vi "GEA3 HEWH Parse ERD.vi"(4 "Enable Heat Pump List":bool, 6 "Enable EMV List?":bool, 8 "Error In":errorcluster, 11 "ERD Data Out":T3[](array[typedef]) {"ERD Number" format="%.0x"}) -> (0 "Error Out":errorcluster, 2 "ERD Data":string[][](array[string]), 3 "ERD Data":T1)   [LabVIEW 2019]
uses:
  type defs/ERD Read Data Out.ctl
  Type Definitions/GEA3 HEWH ERD Data.ctl
  Type Definitions/GEA3 HEWH Mixing Valve.ctl
  library/GEA2_Toolkit.lvlib
panel:
  out "ERD Headers":string[](array[string])=["APPLIANCE SOFTWARE VERSION (0x0100)", "USER SET MODE (0X4020)", "OPERATING MODE (0X4021)", "USER SETPOINT (0x4024)", "ACTUAL SETPOINT (0x4026)", "MODEL DESIGNATOR (0x4042)", "DLB RELAY (0x4068)", "COMPRESSOR RELAY (0x4068)", "LOWER ELEMENT RELAY (0x4068)", "UPPER ELEMENT RELAY (0x4068)", "FAN (0x4068)", "T1 TEMP (0x405F)", "T2 TEMP (0x4060)", "T3A TEMP (0x4061)", "T3B TEMP (0x4062)", "T4 TEMP (0x4063)", "T5 TEMP (0x4064)", "VOLTAGE (0x4066)", "DLB CURRENT (0x4065)", "EEV POSITION (0x4067)", "FLOW EVENTS (0x4069)", "STORED THERMAL CAPACITANCE (0x4058)", "AVAILABLE THERMAL CAPACITANCE (0x4059)", "MAXIMUM THERMAL CAPACITANCE (0X405A)", "NEEA MODE ENABLED (0X404F)", "TANK SIZE (0X4041)", "MIXING VALVE THERMAL CAPACITY SETTING (0X4029)", "T6 TEMP (0x406E)", "T7 TEMP (0x407D)", "MIX VALVE STEP OFFSET (0x4072)", "MIX VALVE STEP ABSOLUTE (0x4073)", "TANK TCO STATE (0x4074)", "OUTLET TCO STATE (0x4075)", "FLOW (0x407E)", "MANUAL (0x407F)", "TANK SETPOINT (0x4078)", "MIX VALVE DELTA T (0x4077)", "PID OUTPUT POSITION (0x407C)", "DAY 1 COLDEST SUPPLY (0x40B0)", "DAY 2 COLDEST SUPPLY (0x40B1)", "DAY 3 COLDEST SUPPLY (0x40B2)", "DAY 4 COLDEST SUPPLY (0x40B3)", "DAY 5 COLDEST SUPPLY (0x40B4)", "DAY 6 COLDEST SUPPLY (0x40B5)", "DAY 7 COLDEST SUPPLY (0x40B6)", "SUPPLY TEMP (0x40B7)", "FIRST STAGE KP GAIN (0xF011)", "FIRST STAGE KI GAIN (0xF012)", "FIRST STAGE KD GAIN (0xF013)", "FIRST STAGE KPQ BITS (0xF014)", "FIRST STAGE KI BITS (0xF015)", "FIRST STAGE KDQ BITS (0xF016)", "SECOND STAGE KP GAIN (0xF021)", "SECOND STAGE KI GAIN (0xF022)", "SECOND STAGE KD GAIN (0xF023)", "SECOND STAGE KPQ BITS (0xF024)", "SECOND STAGE KIQ BITS (0xF025)", "SECOND STAGE KDQ BITS (0xF026)", "THIRD STAGE KP GAIN (0xF031)", "THIRD STAGE KI GAIN (0xF032)", "THIRD STAGE KD GAIN (0xF033)", "THIRD STAGE KPQ BITS (0xF034)", "THIRD STAGE KIQ BITS (0xF035)", "THIRD STAGE KDQ BITS (0xF036)", "FOURTH STAGE KP GAIN (0xF041)", "FOURTH STAGE KI GAIN (0xF042)", "FOURTH STAGE KD GAIN (0xF043)", "FOURTH STAGE KPQ BITS (0xF044)", "FOURTH STAGE KIQ BITS (0xF045)", "FOURTH STAGE KDQ BITS (0xF046)"]
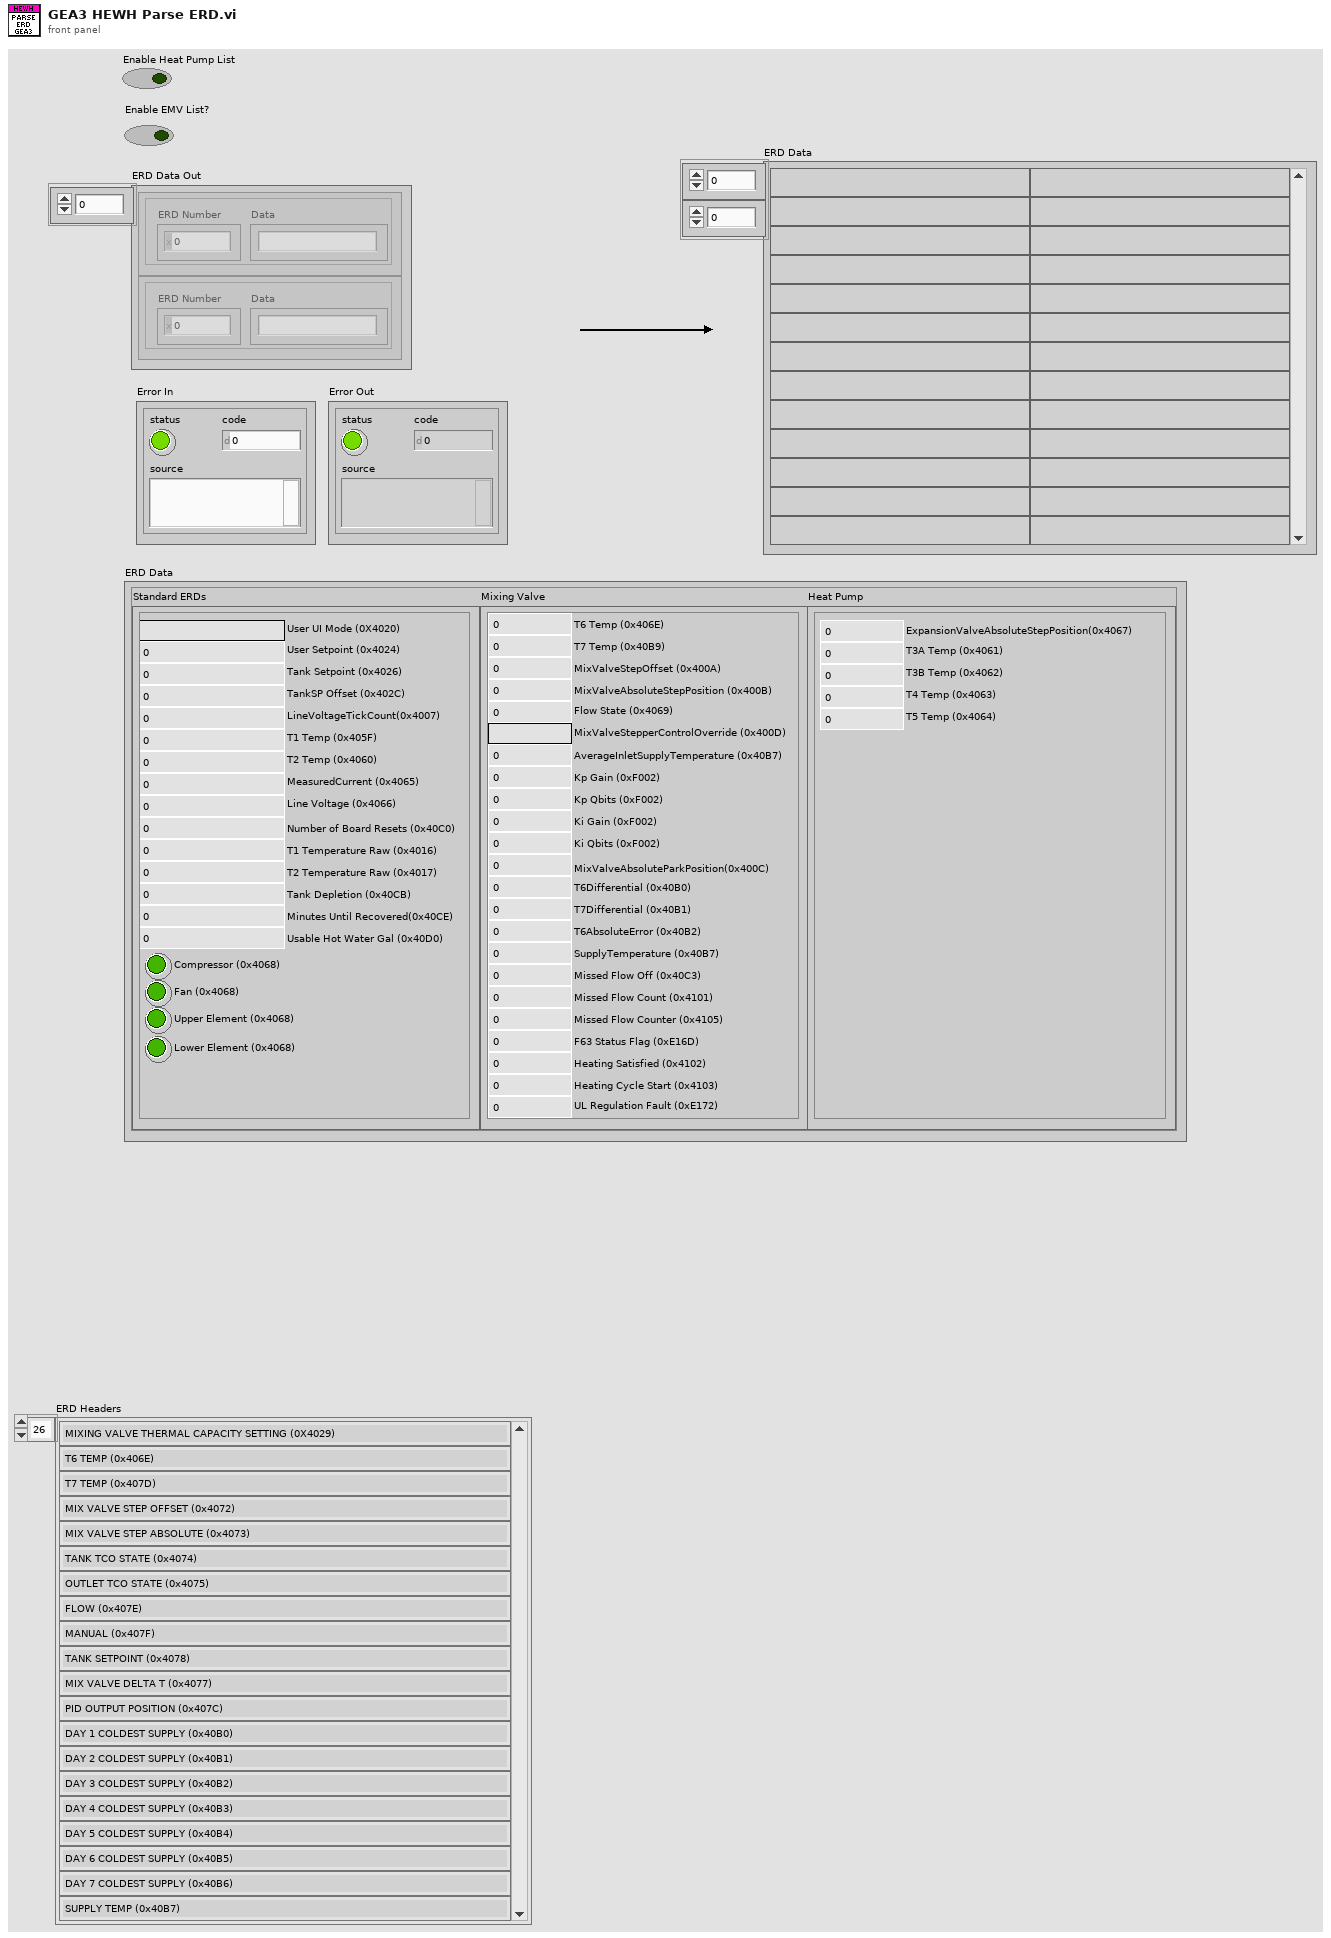
[diagram p1: front panel]
types:
  T1 = typedef "GEA3 HEWH ERD Data.ctl" = cluster{"Mixing Valve":T2, "Standard ERDs":cluster{"User UI Mode (0X4020)":string, "User Setpoint (0x4024)":u16, "TankSP Offset (0x402C)":i16, "Compressor (0x4068)":bool, "Lower Element (0x4068)":bool, "Upper Element (0x4068)":bool, "Fan (0x4068)":bool, "T1 Temp (0x405F)":dbl, "T2 Temp (0x4060)":dbl, "Line Voltage (0x4066)":dbl, "MeasuredCurrent (0x4065)":dbl, "LineVoltageTickCount(0x4007)":u16, "Number of Board Resets (0x40C0)":u16, "T1 Temperature Raw (0x4016)":u16, "T2 Temperature Raw (0x4017)":u16, "Tank Depletion (0x40CB)":u16, "Tank Setpoint (0x4026)":u16, "Minutes Until Recovered(0x40CE)":u16, "Usable Hot Water Gal (0x40D0)":u16}, "Heat Pump":cluster{"ExpansionValveAbsoluteStepPosition(0x4067)":i16, "T3A Temp (0x4061)":dbl, "T3B Temp (0x4062)":dbl, "T4 Temp (0x4063)":dbl, "T5 Temp (0x4064)":dbl}}
  T2 = typedef "GEA3 HEWH Mixing Valve.ctl" = cluster{"T7 Temp (0x40B9)":dbl, "MixValveStepOffset (0x400A)":i16, "MixValveAbsoluteStepPosition (0x400B)":i16, "Flow State (0x4069)":u8, "MixValveStepperControlOverride (0x400D)":string, "AverageInletSupplyTemperature (0x40B7)":dbl, "T6 Temp (0x406E)":dbl, "Kp Gain (0xF002)":u16, "Kp Qbits (0xF002)":u16, "Ki Gain (0xF002)":u16, "Ki Qbits (0xF002)":u16, "MixValveAbsoluteParkPosition(0x400C)":i16, "T7Differential (0x40B1)":dbl, "T6Differential (0x40B0)":dbl, "SupplyTemperature (0x40B7)":dbl, "Missed Flow Off (0x40C3)":u8, "T6AbsoluteError (0x40B2)":dbl, "Missed Flow Count (0x4101)":u16, "Missed Flow Counter (0x4105)":u16, "F63 Status Flag (0xE16D)":u16, "Heating Satisfied (0x4102)":u16, "Heating Cycle Start (0x4103)":u16, "UL Regulation Fault (0xE172)":u8}
  T3 = typedef "GEA2_Toolkit.lvlib/ERD Read Data Out.ctl" = cluster{"ERD Number":u16, "Data":string}
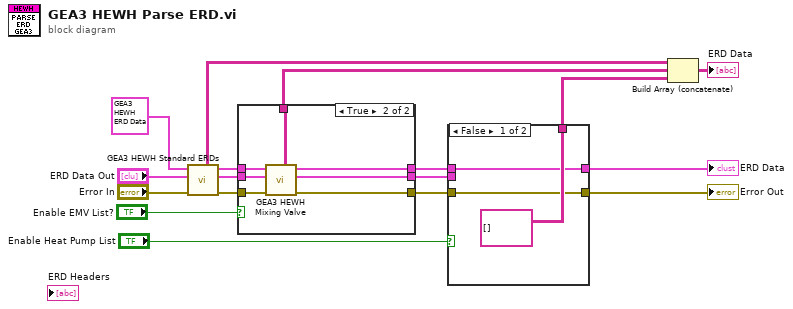
[diagram p0: block diagram]
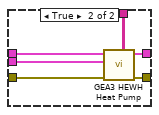
[diagram p2: hidden frame]
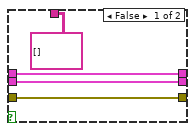
[diagram p3: hidden frame]
diagram:
  n1 = call "GEA3 HEWH Standard ERDs.vi"("Error In"="Error In", "ERD Data Input"="ERD Data Out", "ERD Data  in"=T1 {"Mixing Valve"={"T7 Temp (0x40B9)"=0.0, "MixValveStepOffset (0x400A)"=0, "MixValveAbsoluteStepPosition (0x400B)"=0, "Flow State (0x4069)"=0, "MixValveStepperControlOverride (0x400D)"="", "AverageInletSupplyTemperature (0x40B7)"=0.0, "T6 Temp (0x406E)"=0.0, "Kp Gain (0xF002)"=0, "Kp Qbits (0xF002)"=0, "Ki Gain (0xF002)"=0, "Ki Qbits (0xF002)"=0, "MixValveAbsoluteParkPosition(0x400C)"=0, "T7Differential (0x40B1)"=0.0, "T6Differential (0x40B0)"=0.0, "SupplyTemperature (0x40B7)"=0.0, "Missed Flow Off (0x40C3)"=0, "T6AbsoluteError (0x40B2)"=0.0, "Missed Flow Count (0x4101)"=0, "Missed Flow Counter (0x4105)"=0, "F63 Status Flag (0xE16D)"=0, "Heating Satisfied (0x4102)"=0, "Heating Cycle Start (0x4103)"=0, "UL Regulation Fault (0xE172)"=0}, "Standard ERDs"={"User UI Mode (0X4020)"="", "User Setpoint (0x4024)"=0, "TankSP Offset (0x402C)"=0, "Compressor (0x4068)"=FALSE, "Lower Element (0x4068)"=FALSE, "Upper Element (0x4068)"=FALSE, "Fan (0x4068)"=FALSE, "T1 Temp (0x405F)"=0.0, "T2 Temp (0x4060)"=0.0, "Line Voltage (0x4066)"=0.0, "MeasuredCurrent (0x4065)"=0.0, "LineVoltageTickCount(0x4007)"=0, "Number of Board Resets (0x40C0)"=0, "T1 Temperature Raw (0x4016)"=0, "T2 Temperature Raw (0x4017)"=0, "Tank Depletion (0x40CB)"=0, "Tank Setpoint (0x4026)"=0, "Minutes Until Recovered(0x40CE)"=0, "Usable Hot Water Gal (0x40D0)"=0}, "Heat Pump"={"ExpansionValveAbsoluteStepPosition(0x4067)"=0, "T3A Temp (0x4061)"=0.0, "T3B Temp (0x4062)"=0.0, "T4 Temp (0x4063)"=0.0, "T5 Temp (0x4064)"=0.0}} ("ERD Data")) -> ("Error Out"=w15:errorcluster, "ERD Data Output"=w14:T3[], "ERD Data  out"=w13:T1, "Standard Data"=w10:string[][])  [unwired: 5 in]
  n2 = case shown="True" "Enable EMV List?" {
    tunnel: w15 -> [w20 w28]
    tunnel: w14 -> [w18 w27]
    tunnel: w13 -> [w21 w26]
    tunnel: [w21 w25] -> w6
    tunnel: [w20 w24] -> w5
    tunnel: [string[][] [] ("Mix Valve Data") w23] -> w9
    tunnel: [w18 w22] -> w4
    frame False {
    }
    frame True {
      n3 = call "GEA3 HEWH Mixing Valve.vi"("Error In"=w28, "ERD Data In"=w27, "GEA3 ERD Data"=w26) -> ("Error Out"=w24:errorcluster, "ERD Data Out"=w22:T3[], "GEA3 ERD Data Out"=w25:T1, "Mix Valve Data"=w23:string[][])  [unwired: 5 in]
    }
  }
  n4 = case shown="False" "Enable Heat Pump List" {
    tunnel: w6 -> [w30 w37]
    tunnel: w5 -> [w29 w36]
    tunnel: w4 -> [_ w35]
    tunnel: [string[][] [] ("Mix Valve Data") w34] -> w3
    tunnel: [w30 w33] -> w2
    tunnel: [w29 w32] -> w1
    frame False {
    }
    frame True {
      n5 = call "GEA3 HEWH Heat Pump.vi"("Error In"=w36, "ERD Data Out"=w35, "GEA3 ERD Data"=w37) -> ("Error Out"=w32:errorcluster, "GEA3 ERD Data Out"=w33:T1, "Mix Valve Data"=w34:string[][])  [unwired: 6 in]
    }
  }
  "ERD Data" <- w2
  "Error Out" <- w1
  n6 = Build Array (concatenate)(w10, w9, w3) -> (→"ERD Data":string[][])
